vi "Load Config_Folder Icon Map.vi"(8 "error in (no error)":errorcluster, 10 "Target Folder":path, 11 "Refnum in":T1) -> (0 "error out":errorcluster, 2 "Folder Icon Map":T2, 3 "Refnum out":T1)   [LabVIEW 2019, in "AutoMenuCreator.lvlib"]
doc: "Read all keys from the 'Folder Icons'-section as raw strings and convert them to paths and build a Folder Icon Path Map."
uses:
  AutoMenuCreator.lvlib
  Ctl/Ctl_Config_Folder Icon Map.ctl
  <vilib>/Utility/config.llb/Config Data RefNum.ctl
  <vilib>/Utility/config.llb/NI_LVConfig.lvlib
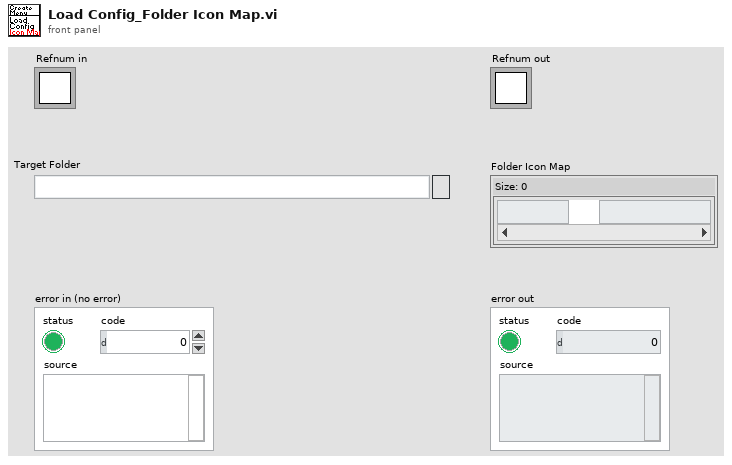
[diagram p1: front panel]
types:
  T1 = typedef "NI_LVConfig.lvlib/Config Data RefNum.ctl" = refnum<k1>
  T2 = typedef "AutoMenuCreator.lvlib/Ctl_Config_Folder Icon Map.ctl" = map{string, path}
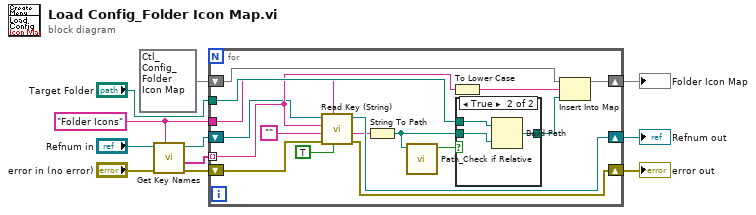
[diagram p0: block diagram]
diagram:
  w8 = "Folder Icons"
  n1 = call <vilib>:"Get Key Names.vi"("section"=w8, "error in (no error)"="error in (no error)", "refnum"="Refnum in") -> ("error out"=w4:errorcluster, "key names"=w9:string[], "refnum out"=w5:T1)  [unwired: 5 in, 1 out]
  n2 = for {
    tunnel: w9 -> [w19] mode=indexing
    tunnel: w8 -> [w18]
    shift-right: [w24] -> w6
    shift-left: T2 {} ("Folder Icon Map") -> [w25]
    shift-right: [w20] -> w1
    shift-left: w4 -> [w21]
    tunnel: "Target Folder" -> [w26]
    shift-right: [w16] -> w2
    shift-left: w5 -> [w17]
    n3 = call <vilib>:"Read Key (String).vi"("read raw string? (F)"=TRUE, "section"=w18, "error in (no error)"=w21, "default value"="", "key"=w19, "refnum"=w17) -> ("error out"=w20:errorcluster, "value"=w14:string, "refnum out"=w16:T1)  [unwired: 2 in, 1 out]
    n4 = String To Path(string=w14) -> (path=w13:path)
    n5 = call "Path_Check if Relative.vi"("Path"=w13) -> ("Relative Path?"=w27:bool)  [unwired: 10 in]
    n6 = To Lower Case(string=w19) -> (all lower case string=w22:string)
    n7 = case shown="True" w27 {
      tunnel: w26 -> [_ w31]
      tunnel: w13 -> [w28 w30]
      tunnel: [w28 w29] -> w23
      frame False {
      }
      frame True {
        n8 = Build Path(base path=w31, name or relative path=w30) -> (appended path=w29:path)
      }
    }
    n9 = Insert Into Map(map in=w25, key=w22, value=w23) -> (map out=w24:T2)  [unwired: 2 out]
  }
  "Folder Icon Map" <- w6
  "error out" <- w1
  "Refnum out" <- w2
